vi "Viewer_TopLevel_1.vi"() -> ()   [LabVIEW 2009]
doc: "Use this template to create an application that executes until you click the Stop button. Unlike the Single Loop Application VI that uses polling, this VI uses the Event Structure."
uses:
  <vilib>/Utility/file.llb/Read From Spreadsheet File (DBL).vi
  <vilib>/Utility/file.llb/Read From Spreadsheet File (string).vi
panel:
  out "XY Graph":cluster{"Y":dbl[], "Y":dbl[]}[](graph)
  out "All Files in Dir":path[](array[path])
  out "Intensity Graph":dbl[][](graph)
  in  "open":bool
  in  "Path":path
  in  "stop":bool
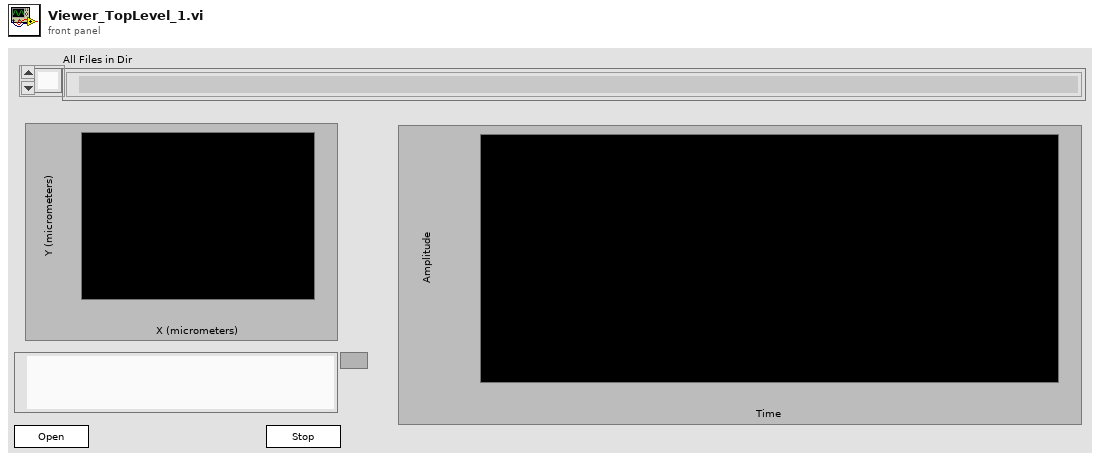
[diagram p1: front panel]
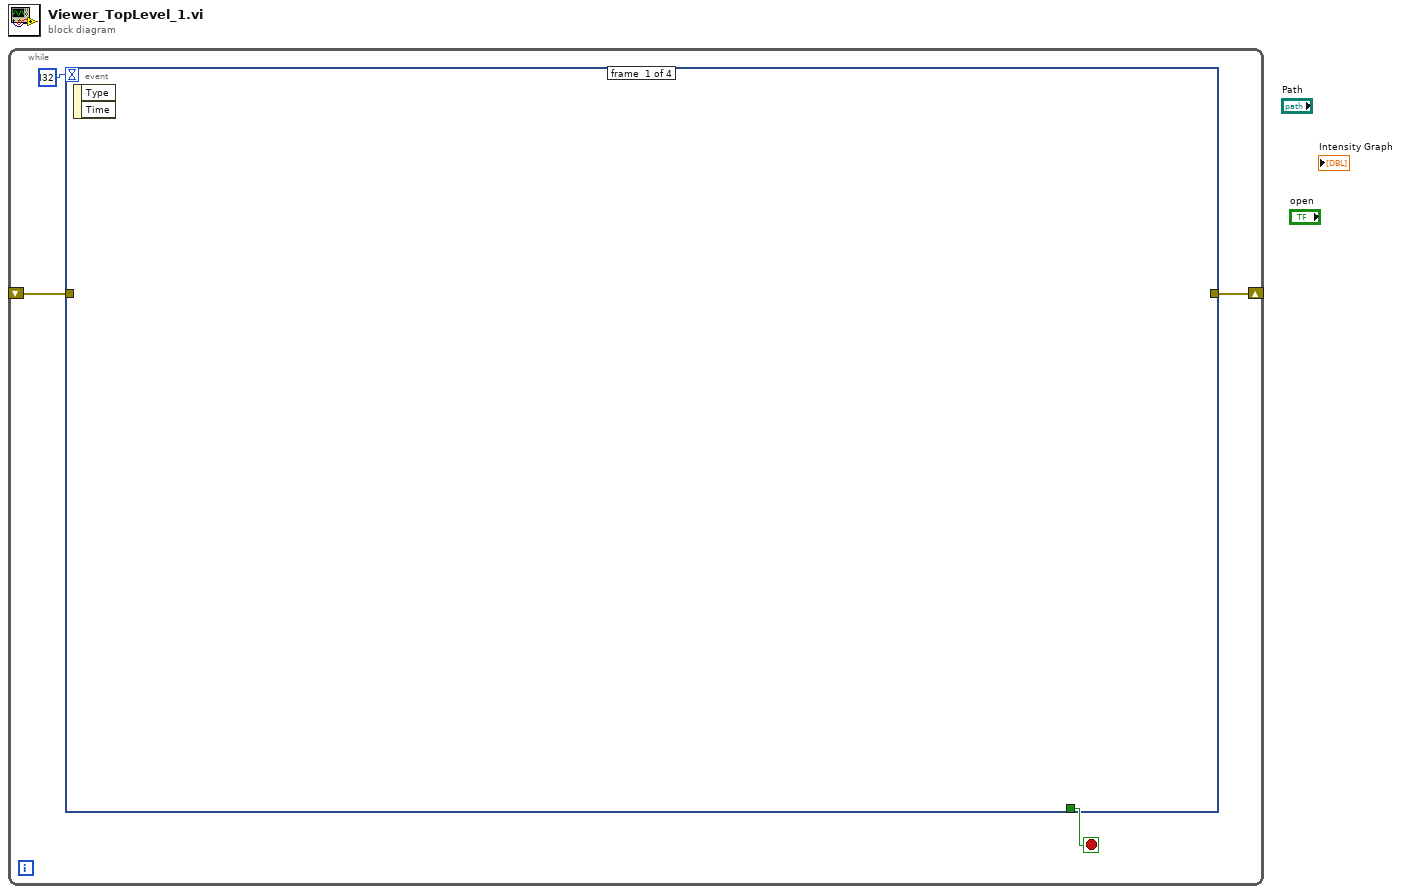
[diagram p0: block diagram]
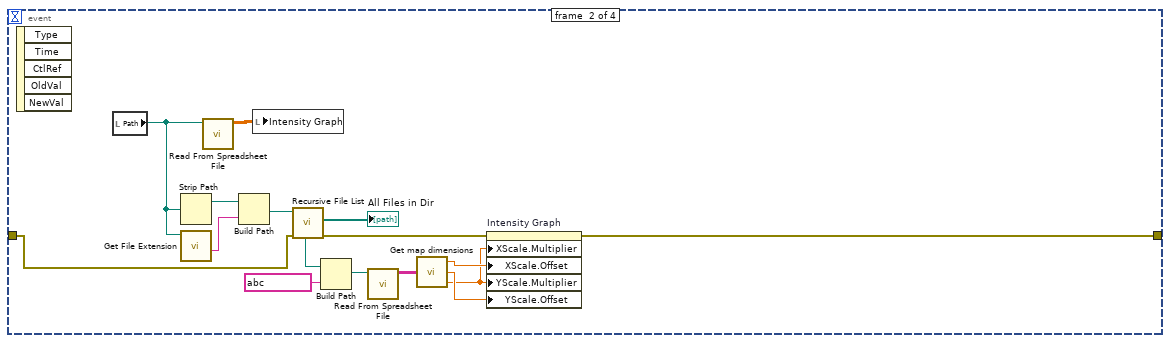
[diagram p2: hidden frame]
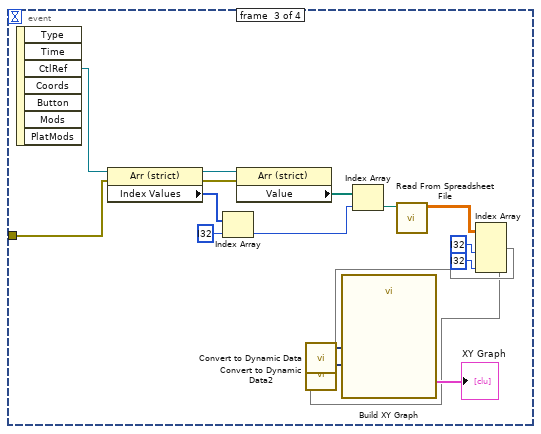
[diagram p3: hidden frame]
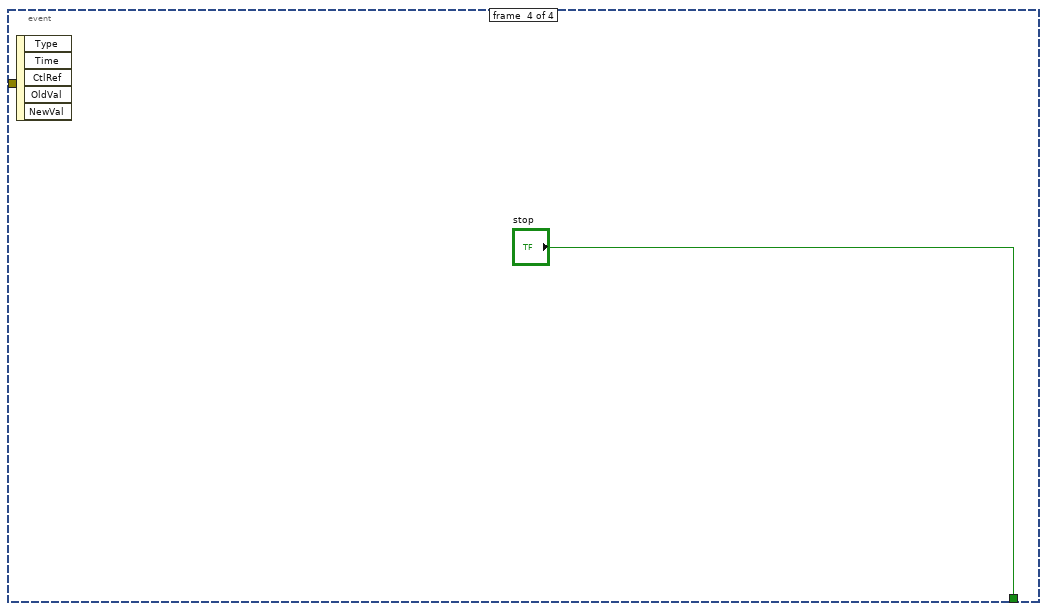
[diagram p4: hidden frame]
diagram:
  n1 = while {
    shift-right: [w3] -> _
    shift-left: _ -> [w2]
    stop <- w4 stop-if-true
    n2 = event shown="[1] \"open\": Value Change" {
      selector: _ -> [_ _ _ _]
      dyn-events: _ -> [_ _ _ _]
      timeout: i32 ? -> [_ _ _ _]
      tunnel: [_ _ _ "stop"] -> w4
      tunnel: [_ w8 _ _] -> w3
      tunnel: w2 -> [_ w15 w35 _]
      event #0 {
        n3 = event-data() -> ()  [unwired: 1 in, 2 out]
      }
      event #1 {
        n4 = event-data() -> ()  [unwired: 1 in, 5 out]
        n5 = local read "Path"() -> (w18:path)
        n6 = Strip Path(path=w18) -> (stripped path=w17:path)  [unwired: 1 out]
        n7 = call <vilib>:"Get File Extension.vi"("file"=w18) -> ("filename without extension"=w19:string)  [unwired: 7 in, 3 out]
        n8 = call-poly <vilib>:"Read From Spreadsheet File.vi"("file path (dialog if empty)"=w18) -> ("all rows"=w16:dbl[][])  [unwired: 6 in, 4 out]
        n9 = Build Path(base path=w17, name or relative path=w19) -> (appended path=w13:path)
        n10 = local write "Intensity Graph"(w16) -> ()
        n11 = call <vilib>:"Recursive File List.vi"("error in (no error)"=w15, "Folder Path"=w13) -> ("error out"=w9:errorcluster, "All Files in Dir"=→"All Files in Dir":path[])  [unwired: 5 in, 3 out]
        n12 = Build Path(base path=w13, name or relative path=string ?) -> (appended path=w11:path)
        n13 = call-poly <vilib>:"Read From Spreadsheet File.vi"("file path (dialog if empty)"=w11) -> ("all rows"=w10:string[][])  [unwired: 6 in, 4 out]
        n14 = call "Get map dimensions.vi"("all rows"=w10) -> ("Step"=w5:dbl, "Y0"=w6:dbl, "X0"=w7:dbl)
        n15 = property on="Intensity Graph" class="IntGraph (strict)"(error in=w9, "XScale.Multiplier"=w5, "XScale.Offset"=w7, "YScale.Multiplier"=w5, "YScale.Offset"=w6) -> (error out=w8:errorcluster)  [unwired: 1 in, 1 out]
      }
      event #2 {
        n16 = event-data() -> ("CtlRef"=w36:refnum<vi>)  [unwired: 1 in, 6 out]
        n17 = property on="Property Node" class="Arr (strict)"(reference=w36, error in=w35) -> (reference out=w32:refnum<vi>, error out=w31:errorcluster, "Index Values"=w33:u32[])
        n18 = Index Array(array=w33, index=i32 ?) -> (element=w29:u32)
        n19 = property class="Arr (strict)"(reference=w32, error in=w31) -> ("Value"=w30:path[])  [unwired: 2 out]
        n20 = Index Array(array=w30, index=w29) -> (element=w28:path)
        n21 = call-poly <vilib>:"Read From Spreadsheet File.vi"("file path (dialog if empty)"=w28) -> ("all rows"=w27:dbl[][])  [unwired: 6 in, 4 out]
        n22 = Index Array(array=w27, index (col) #1=i32 ? ("index (row)"), index (col) #2=i32 ? ("index (row)")) -> (element #1=w25:dbl[], element #2=w23:dbl[])  [unwired: 2 in]
        n23 = call "Convert to Dynamic Data"("Array"=w25) -> ("Dynamic Data Type"=w24:dynamicdata)  [unwired: 3 in]
        n24 = call "Convert to Dynamic Data2"("Array"=w23) -> ("Dynamic Data Type"=w22:dynamicdata)  [unwired: 3 in]
        n25 = call "Build XY Graph"("Y Input"=w22, "X Input"=w24) -> ("XY Graph"=→"XY Graph":cluster{"Y":dbl[], "Y":dbl[]}[])  [unwired: 3 in, 6 out]
      }
      event #3 {
        n26 = event-data() -> ()  [unwired: 1 in, 5 out]
      }
    }
  }
